vi "Write RP Level Configuration.vi"(8 "error in (no error)":errorcluster, 10 "RP Delayed Configuration":T1={"Pre-trigger duration"=0.01, "Post-trigger duration"=0.1, "Rate"=1000000.0, "Ranges"=[10.0], "Re-name channels"=[], "Active channels"="0:1", "External clock"=FALSE, "Output delay"=0.1, "Raising edge "=FALSE, "Trigger level"=0.001} {"Trigger level" format="%#_6pV"; "Output delay" format="%#_6ps"; "Rate" format="%#_8pHz"; "Post-trigger duration" format="%#_6ps"; "Pre-trigger duration" format="%#_6ps"; "Ranges" format="%#_6pV"}, 11 "RP Delayed in":refnum<class "RP Level.lvclass">) -> (0 "error out":errorcluster, 3 "RP Delayed out":refnum<class "RP Level.lvclass">)   [LabVIEW 2018, in "RP Level.lvclass"]
uses:
  RP Level.lvclass
  C:/github/LabActor/Template Module/Template Module.lvclass
  NHMFL_Core/Libraries/Red Pitaya/RP Level Configuration.ctl
  Template Module/Template Module.lvclass/Template Module.ctl
  Template Module/Write Configuration.vi
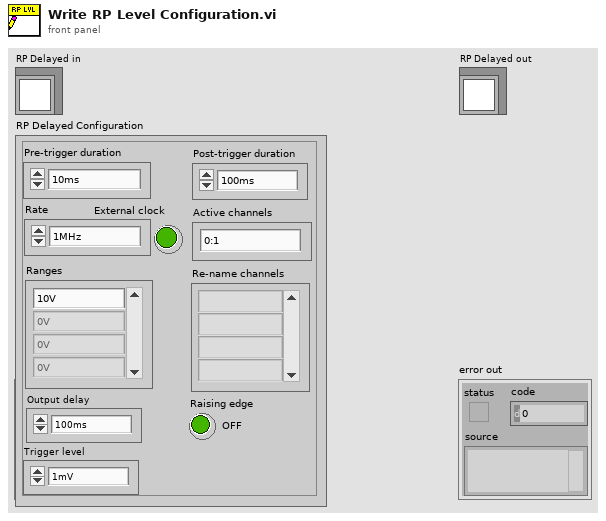
[diagram p1: front panel]
types:
  T1 = typedef "RP Level Configuration.ctl" = cluster{"Pre-trigger duration":dbl, "Post-trigger duration":dbl, "Rate":dbl, "Ranges":dbl[], "Re-name channels":string[], "Active channels":string, "External clock":bool, "Output delay":dbl, "Raising edge ":bool, "Trigger level":dbl}
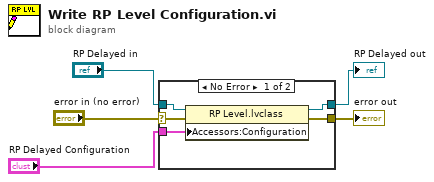
[diagram p0: block diagram]
diagram:
  n1 = case shown="No Error" "error in (no error)" {
    selector: "error in (no error)" -> [w10 w11]
    tunnel: [w9 w11] -> w4
    tunnel: [w7 w12] -> w2
    tunnel: "RP Delayed in" -> [w8 w12]
    tunnel: "RP Delayed Configuration" -> [w6 _]
    frame No Error {
      n2 = property class="RP Level.lvclass"(reference=w8, error in=w10, "Accessors:Configuration"=w6) -> (reference out=w7:refnum<class "RP Level.lvclass">, error out=w9:errorcluster)
    }
    frame Error {
    }
  }
  "error out" <- w4
  "RP Delayed out" <- w2
